vi "Make_Body_Test.vi"() -> ()   [LabVIEW 2016]
panel:
  out "data string":string
  out "output array 2":u8[](array[numeric])
  out "spreadsheet string":string
  out "output array":u8[](array[numeric]) format="%02x"
  out "Before Checksum":u8[](array[numeric])
  out "Array":u8[](array[numeric])
  in  "error out":errorcluster
  out "P2":u32 format="%x"
  in  "Target Devices":T1={"P1 Cluster"={"P1_D1"=TRUE, "P1_D2"=TRUE, "P1_D3"=TRUE, "P1_D4"=TRUE, "P1_D5"=TRUE, "P1_D6"=TRUE, "P1_D7"=TRUE, "P1_D8"=TRUE, "P1_D9"=TRUE, "P1_D10"=TRUE, "P1_D11"=TRUE, "P1_D12"=TRUE, "P1_D13"=TRUE, "P1_D14"=TRUE, "P1_D15"=TRUE, "P1_D16"=TRUE, "P1_D17"=TRUE, "P1_D18"=TRUE, "P1_D19"=TRUE, "P1_D20"=TRUE, "P1_D21"=TRUE, "P1_D22"=TRUE, "P1_D23"=TRUE, "P1_D24"=TRUE}, "P2 Cluster"={"P2_D1"=TRUE, "P2_D2"=TRUE, "P2_D3"=TRUE, "P2_D4"=TRUE, "P2_D5"=TRUE, "P2_D6"=TRUE, "P2_D7"=TRUE, "P2_D8"=TRUE, "P2_D9"=TRUE, "P2_D10"=TRUE, "P2_D11"=TRUE, "P2_D12"=TRUE, "P2_D13"=TRUE, "P2_D14"=TRUE, "P2_D15"=TRUE, "P2_D16"=TRUE, "P2_D17"=TRUE, "P2_D18"=TRUE, "P2_D19"=TRUE, "P2_D20"=TRUE, "P2_D21"=TRUE, "P2_D22"=TRUE, "P2_D23"=TRUE, "P2_D24"=TRUE}}
  in  "Target String":string="{1:24,1:24,[],[]}"
  in  "Update Targets":bool
  out "P1":u32 format="%x"
  out "Header array":u8[](array[numeric])
  # "P2"
  # "P1"
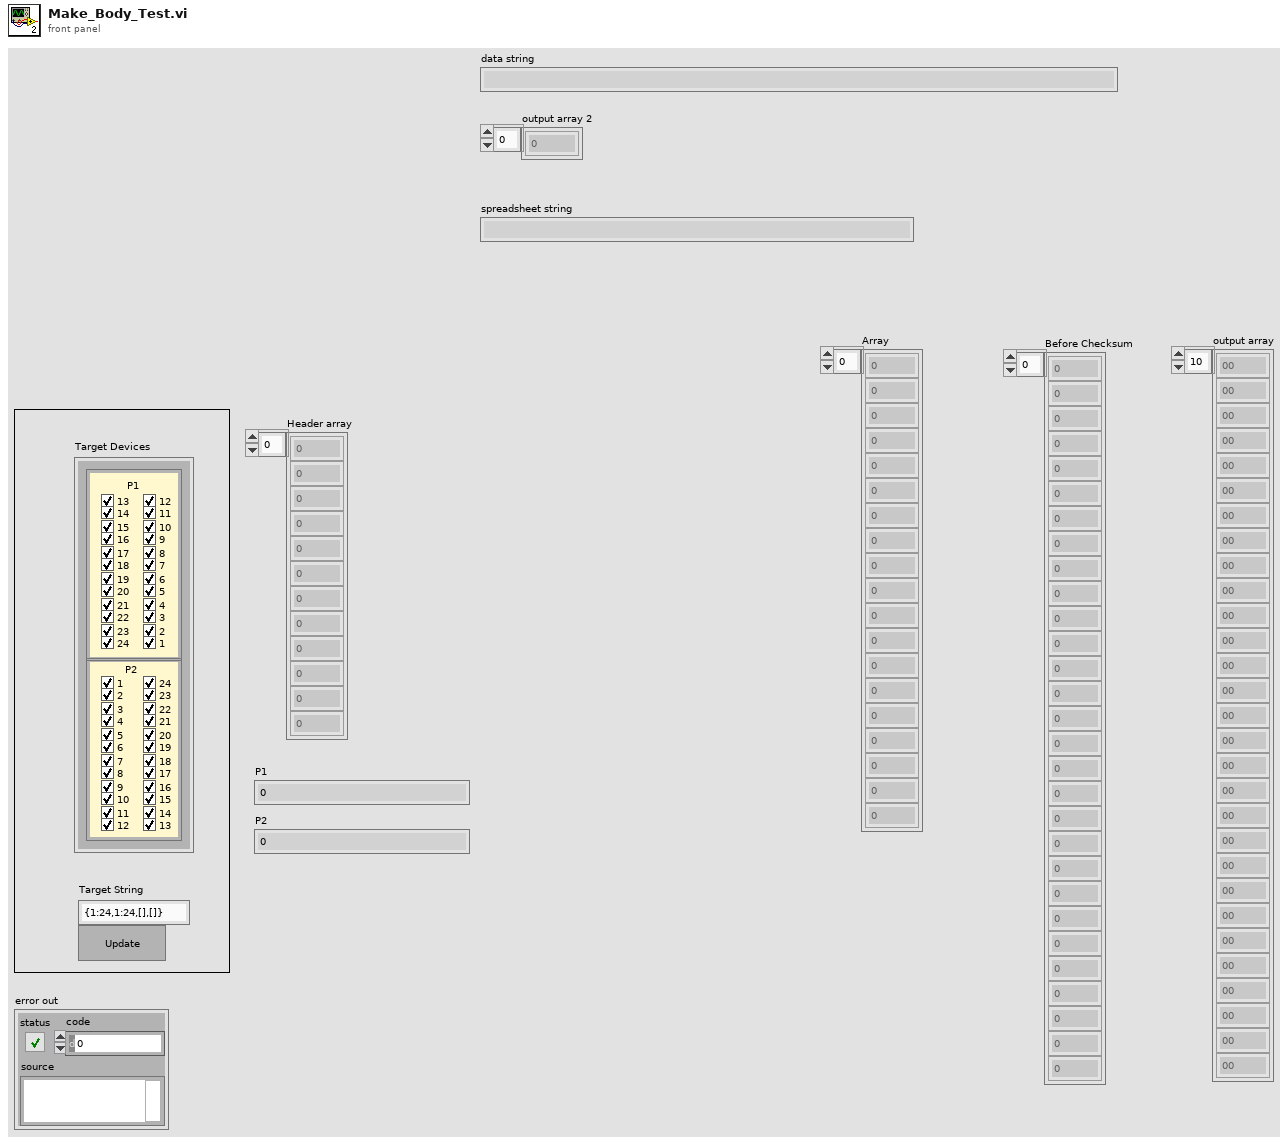
[diagram p1: front panel]
types:
  T1 = cluster{"P1 Cluster":cluster{"P1_D1":bool, "P1_D2":bool, "P1_D3":bool, "P1_D4":bool, "P1_D5":bool, "P1_D6":bool, "P1_D7":bool, "P1_D8":bool, "P1_D9":bool, "P1_D10":bool, "P1_D11":bool, "P1_D12":bool, "P1_D13":bool, "P1_D14":bool, "P1_D15":bool, "P1_D16":bool, "P1_D17":bool, "P1_D18":bool, "P1_D19":bool, "P1_D20":bool, "P1_D21":bool, "P1_D22":bool, "P1_D23":bool, "P1_D24":bool}, "P2 Cluster":cluster{"P2_D1":bool, "P2_D2":bool, "P2_D3":bool, "P2_D4":bool, "P2_D5":bool, "P2_D6":bool, "P2_D7":bool, "P2_D8":bool, "P2_D9":bool, "P2_D10":bool, "P2_D11":bool, "P2_D12":bool, "P2_D13":bool, "P2_D14":bool, "P2_D15":bool, "P2_D16":bool, "P2_D17":bool, "P2_D18":bool, "P2_D19":bool, "P2_D20":bool, "P2_D21":bool, "P2_D22":bool, "P2_D23":bool, "P2_D24":bool}}
  T2 = cluster{"P1_D1":bool, "P1_D2":bool, "P1_D3":bool, "P1_D4":bool, "P1_D5":bool, "P1_D6":bool, "P1_D7":bool, "P1_D8":bool, "P1_D9":bool, "P1_D10":bool, "P1_D11":bool, "P1_D12":bool, "P1_D13":bool, "P1_D14":bool, "P1_D15":bool, "P1_D16":bool, "P1_D17":bool, "P1_D18":bool, "P1_D19":bool, "P1_D20":bool, "P1_D21":bool, "P1_D22":bool, "P1_D23":bool, "P1_D24":bool}
  T3 = cluster{"P2_D1":bool, "P2_D2":bool, "P2_D3":bool, "P2_D4":bool, "P2_D5":bool, "P2_D6":bool, "P2_D7":bool, "P2_D8":bool, "P2_D9":bool, "P2_D10":bool, "P2_D11":bool, "P2_D12":bool, "P2_D13":bool, "P2_D14":bool, "P2_D15":bool, "P2_D16":bool, "P2_D17":bool, "P2_D18":bool, "P2_D19":bool, "P2_D20":bool, "P2_D21":bool, "P2_D22":bool, "P2_D23":bool, "P2_D24":bool}
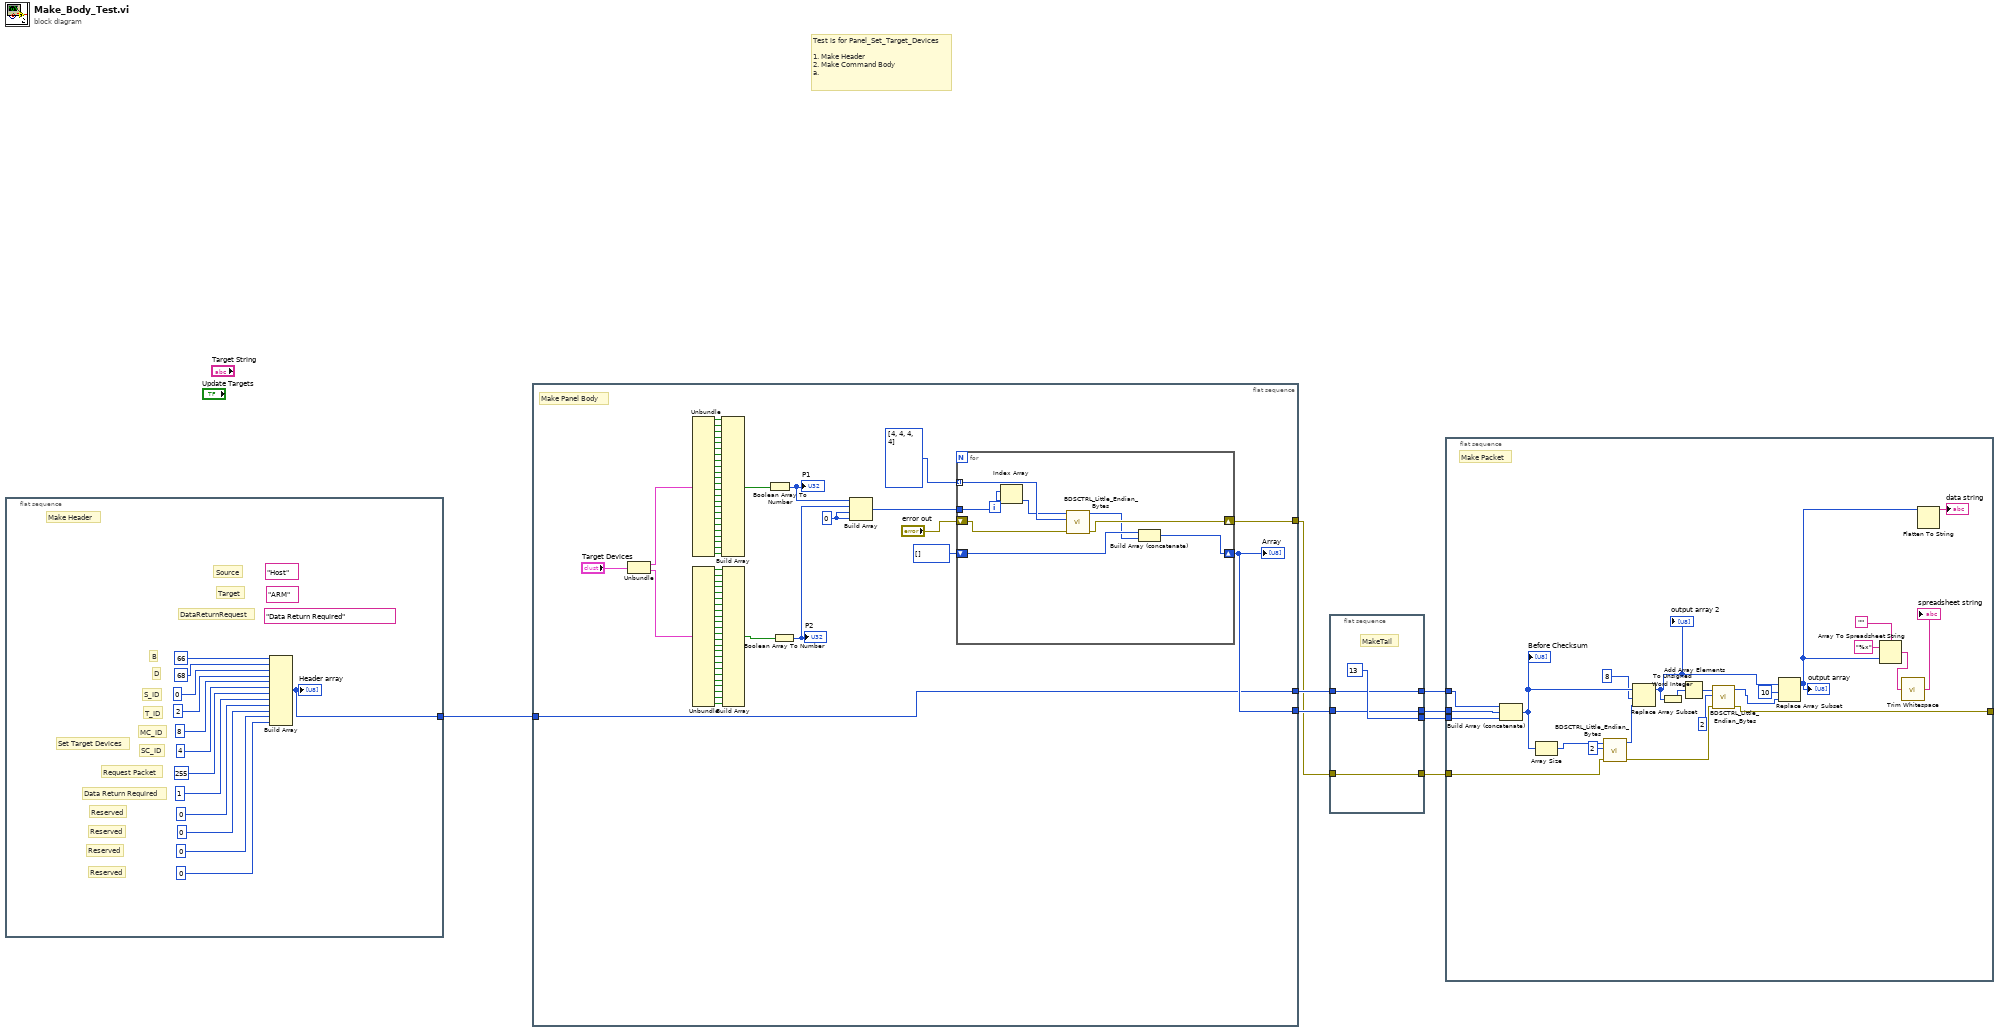
[diagram p0: block diagram]
diagram:
  # "Test is for Panel_Set_Target_Devices\n\n1. Make Header\n2. Make Command Body\na."
  n1 = flat-sequence {
    tunnel: [w9] -> w8
    frame #0 {
      (unwired) "Data Return Required"
      (unwired) "ARM"
      (unwired) "Host"
      # "Make Header"
      # "D"
      # "B"
      # "Set Target Devices"
      # "Reserved"
      # "Reserved"
      # "Reserved"
      # "Reserved"
      # "Data Return Required"
      # "Request Packet"
      # "SC_ID"
      # "MC_ID"
      # "T_ID"
      # "S_ID"
      # "DataReturnRequest"
      # "Target"
      # "Source"
      n2 = Build Array(u8 66, u8 68, u8 0, u8 2, u8 8, u8 4, u8 255, u8 1, u8 0, u8 0, u8 0, u8 0) -> (w9:u8[])
      "Header array" <- w9
    }
  }
  n3 = flat-sequence {
    tunnel: w8 -> [w23]
    tunnel: [w24] -> w5
    tunnel: [w23] -> w4
    tunnel: [w22] -> w2
    frame #0 {
      w29 = u32 0
      # "Make Panel Body"
      n4 = Unbundle("Target Devices") -> ("P1 Cluster"=w34:T2, "P2 Cluster"=w35:T3)
      n5 = Unbundle(w34) -> ("P1_D1"=w36:bool, "P1_D2"=w37:bool, "P1_D3"=w38:bool, "P1_D4"=w39:bool, "P1_D5"=w40:bool, "P1_D6"=w41:bool, "P1_D7"=w42:bool, "P1_D8"=w43:bool, "P1_D9"=w44:bool, "P1_D10"=w45:bool, "P1_D11"=w46:bool, "P1_D12"=w47:bool, "P1_D13"=w48:bool, "P1_D14"=w49:bool, "P1_D15"=w50:bool, "P1_D16"=w51:bool, "P1_D17"=w52:bool, "P1_D18"=w53:bool, "P1_D19"=w54:bool, "P1_D20"=w55:bool, "P1_D21"=w56:bool, "P1_D22"=w57:bool, "P1_D23"=w58:bool, "P1_D24"=w59:bool)
      n6 = Unbundle(w35) -> ("P2_D1"=w60:bool, "P2_D2"=w61:bool, "P2_D3"=w62:bool, "P2_D4"=w63:bool, "P2_D5"=w64:bool, "P2_D6"=w65:bool, "P2_D7"=w66:bool, "P2_D8"=w67:bool, "P2_D9"=w68:bool, "P2_D10"=w69:bool, "P2_D11"=w70:bool, "P2_D12"=w71:bool, "P2_D13"=w72:bool, "P2_D14"=w73:bool, "P2_D15"=w74:bool, "P2_D16"=w75:bool, "P2_D17"=w76:bool, "P2_D18"=w77:bool, "P2_D19"=w78:bool, "P2_D20"=w79:bool, "P2_D21"=w80:bool, "P2_D22"=w81:bool, "P2_D23"=w82:bool, "P2_D24"=w83:bool)
      n7 = Build Array(w36, w37, w38, w39, w40, w41, w42, w43, w44, w45, w46, w47, w48, w49, w50, w51, w52, w53, w54, w55, w56, w57, w58, w59) -> (w84:bool[])
      n8 = Build Array(w60, w61, w62, w63, w64, w65, w66, w67, w68, w69, w70, w71, w72, w73, w74, w75, w76, w77, w78, w79, w80, w81, w82, w83) -> (w32:bool[])
      n9 = Boolean Array To Number(Boolean array=w84) -> (number=w31:u32)
      "P1" <- w31
      n10 = Boolean Array To Number(Boolean array=w32) -> (number=w30:u32)
      "P2" <- w30
      n11 = Build Array(w31, w30, w29, w29) -> (w28:u32[])
      n12 = for {
        tunnel: w28 -> [w91]
        tunnel: u8[] [4, 4, 4, 4] -> [w93] mode=indexing
        shift-right: [w90] -> w24
        shift-left: u8[] [] -> [w87]
        shift-right: [w89] -> w22
        shift-left: "error out" -> [w88]
        i -> [w92]
        n13 = Index Array(array=w91, index=w92) -> (element=w85:u32)
        n14 = call "BDSCTRL_Little_Endian_Bytes.vi"("error in"=w88, "Number of Bytes"=w93, "Value"=w85) -> ("error out"=w89:errorcluster, "Hex array"=w86:u8[])  [unwired: 7 in]
        n15 = Build Array (concatenate)(w87, w86) -> (w90:u8[])
      }
      "Array" <- w24
    }
  }
  n16 = flat-sequence {
    tunnel: [u8 13] -> w7
    tunnel: [w96] -> w6
    tunnel: w5 -> [w96]
    tunnel: w4 -> [w95]
    tunnel: [w95] -> w3
    tunnel: w2 -> [w94]
    tunnel: [w94] -> w1
    frame #0 {
      # "MakeTail"
    }
  }
  n17 = flat-sequence {
    tunnel: w7 -> [w120]
    tunnel: w6 -> [w119]
    tunnel: w3 -> [w118]
    tunnel: w1 -> [w115]
    tunnel: [w107] -> _
    frame #0 {
      # "Make Packet"
      n18 = Build Array (concatenate)(w118, w119, w120) -> (w114:u8[])
      "Before Checksum" <- w114
      n19 = Array Size(array=w114) -> (size(s)=w117:i32)
      n20 = call "BDSCTRL_Little_Endian_Bytes.vi"("error in"=w115, "Number of Bytes"=u8 2, "Value"=w117) -> ("error out"=w110:errorcluster, "Hex array"=w112:u8[])  [unwired: 7 in]
      n21 = Replace Array Subset(array=w114, new element=w112, index=8) -> (w102:u8[])
      "output array 2" <- w102
      n22 = To Unsigned Word Integer(number=w102) -> (unsigned 16bit integer=w101:u16[])
      n23 = Add Array Elements(numeric array=w101) -> (sum=w100:u16)
      n24 = call "BDSCTRL_Little_Endian_Bytes.vi"("error in"=w110, "Number of Bytes"=u8 2, "Value"=w100) -> ("error out"=w107:errorcluster, "Hex array"=w108:u8[])  [unwired: 7 in]
      n25 = Replace Array Subset(array=w102, new element=w108, index=10) -> (w99:u8[])
      "output array" <- w99
      n26 = Array To Spreadsheet String(delimiter (Tab)="", array=w99, 3:"%x" ("format string")) -> (spreadsheet string=w104:string)
      n27 = call <vilib>:"Trim Whitespace.vi"("string"=w104) -> ("trimmed string"=→"spreadsheet string":string)  [unwired: 1 in]
      n28 = Flatten To String(anything=w99) -> (data string=→"data string":string)  [unwired: 3 in, 2 out]
    }
  }
